vi "UNIX_Time.vi"(8 "error in (no error)":errorcluster) -> (0 "error out":errorcluster, 1 "Time zones addition":u32, 2 "Daylight savings subtraction":u32, 3 "Unix time - UTC":u32)   [LabVIEW 2013]
doc: "Outputs the current UNIX time (converts from the 1904 epoch LabVIEW based time to the 1970 UNIX epoch time). In addition, this VI takes into account the current time zone (and daylight saving settings) you have on your computer to get the accurate UNIX time conversion."
uses:
  kernel32.dll
panel:
  out "Timezoneinfotype":i32
  out "Sample UTC calc":u32
  out "Local time stamp":timestamp
  # "Seconds since midnight Jan 1st, 1970\nin UTC/GMT time"
  # "Hours"
  # "Hours"
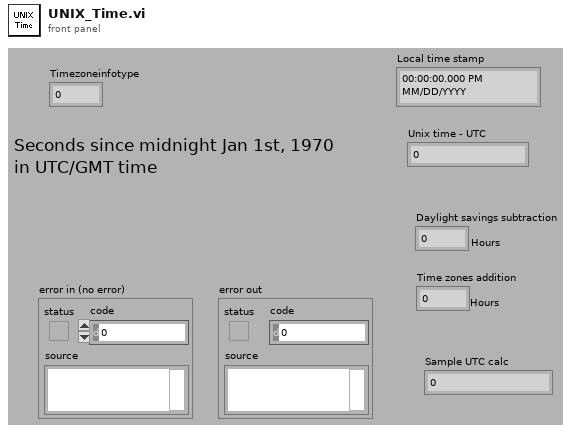
[diagram p1: front panel]
types:
  T1 = cluster{"[0]":u16, "[1]":u16, "[2]":u16, "[3]":u16, "[4]":u16, "[5]":u16, "[6]":u16, "[7]":u16, "[8]":u16, "[9]":u16, "[10]":u16, "[11]":u16, "[12]":u16, "[13]":u16, "[14]":u16, "[15]":u16, "[16]":u16, "[17]":u16, "[18]":u16, "[19]":u16, "[20]":u16, "[21]":u16, "[22]":u16, "[23]":u16, "[24]":u16, "[25]":u16, "[26]":u16, "[27]":u16, "[28]":u16, "[29]":u16, "[30]":u16, "[31]":u16, "[32]":u16, "[33]":u16, "[34]":u16, "[35]":u16, "[36]":u16, "[37]":u16, "[38]":u16, "[39]":u16, "[40]":u16, "[41]":u16, "[42]":u16, "[43]":u16, "[44]":u16, "[45]":u16, "[46]":u16, "[47]":u16, "[48]":u16, "[49]":u16, "[50]":u16, "[51]":u16, "[52]":u16, "[53]":u16, "[54]":u16, "[55]":u16, "[56]":u16, "[57]":u16, "[58]":u16, "[59]":u16, "[60]":u16, "[61]":u16, "[62]":u16, "[63]":u16, "[64]":u16, "[65]":u16, "[66]":u16, "[67]":u16, "[68]":u16, "[69]":u16, "[70]":u16, "[71]":u16, "[72]":u16, "[73]":u16, "[74]":u16, "[75]":u16, "[76]":u16, "[77]":u16, "[78]":u16, "[79]":u16, "[80]":u16, "[81]":u16, "[82]":u16, "[83]":u16, "[84]":u16, "[85]":u16}
  T2 = typedef "LVDateTimeRec.ctl" = cluster{"fractional second":dbl, "second":i32, "minute":i32, "hour":i32, "day of month":i32, "month":i32, "year":i32, "day of week":i32, "day of year":i32, "DST":i32}
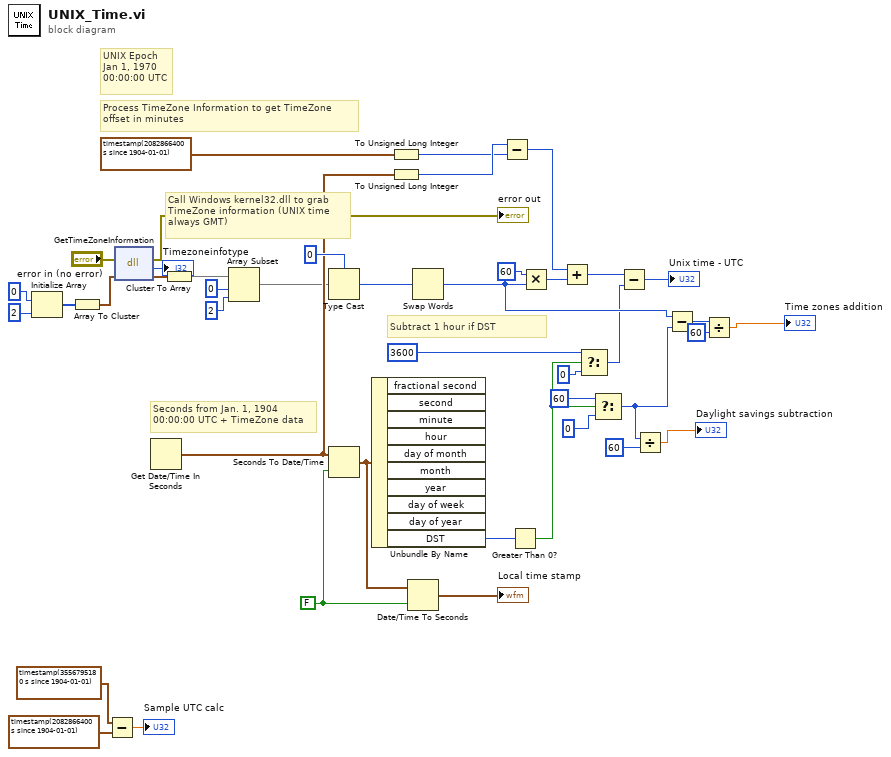
[diagram p0: block diagram]
diagram:
  w24 = FALSE ("to UTC (F)")
  # "Subtract 1 hour if DST"
  # "Seconds from Jan. 1, 1904\n00:00:00 UTC + TimeZone data"
  # "UNIX Epoch\nJan 1, 1970\n00:00:00 UTC"
  # "Process TimeZone Information to get TimeZone\noffset in minutes"
  # "Call Windows kernel32.dll to grab\nTimeZone information (UNIX time\nalways GMT)"
  n1 = Initialize Array(u16 0 ("element"), 2 ("dimension size")) -> (w40:u16[])
  n2 = Array To Cluster(array=w40) -> (cluster=w37:T1)
  n3 = Subtract(x=timestamp(3556795180 s since 1904-01-01), y=timestamp(2082866400 s since 1904-01-01)) -> (x-y=→"Sample UTC calc":dbl)
  n4 = dll-call lib="kernel32.dll" fn="GetTimeZoneInformation"(error in="error in (no error)", "lpTimeZoneInformation"=w37) -> (error out=→"error out":errorcluster, "return type"=→"Timezoneinfotype":i32, "lpTimeZoneInformation"=w36:T1)  [unwired: 2 in, 1 out]
  n5 = Get Date/Time In Seconds() -> (seconds since 1Jan1904=w20:timestamp)
  n6 = Cluster To Array(cluster=w36) -> (array=w35:u16[])
  n7 = Array Subset(array=w35, index=0, length=2) -> (w12:u16[])
  n8 = Type Cast(type=0, x=w12) -> (*(type *) &x=w31:i32)
  n9 = Seconds To Date/Time(time stamp (now)=w20, to UTC (F)=w24) -> (date time rec=w23:T2)
  n10 = Unbundle By Name(w23) -> ("DST"=w19:i32)  [unwired: 9 out]
  n11 = To Unsigned Long Integer(number=timestamp(2082866400 s since 1904-01-01)) -> (unsigned 32bit integer=w41:u32)
  n12 = To Unsigned Long Integer(number=w20) -> (unsigned 32bit integer=w42:u32)
  n13 = Date/Time To Seconds(1:w24, 2:w23) -> (0:→"Local time stamp":timestamp)
  n14 = Swap Words(1:w31) -> (0:w11:i32)
  n15 = Subtract(x=w42, y=w41) -> (x-y=w30:u32)
  n16 = Greater Than 0?(x=w19) -> (x > 0?=w9:bool)
  n17 = Multiply(x=u32 60 ("y"), y=w11) -> (x*y=w29:u32)
  n18 = Add(x=w30, y=w29) -> (x+y=w15:u32)
  n19 = Select(t=u32 3600, s=w9, f=u32 0) -> (s? t:f=w10:u32)
  n20 = Select(t=u32 60 ("f"), s=w9, f=u32 0) -> (s? t:f=w3:u32)
  n21 = Subtract(x=w15, y=w10) -> (x-y=→"Unix time - UTC":u32)
  n22 = Divide(x=w3, y=u32 60) -> (x/y=→"Daylight savings subtraction":dbl)
  n23 = Subtract(x=w11, y=w3) -> (x-y=w6:u32)
  n24 = Divide(x=w6, y=u32 60) -> (x/y=→"Time zones addition":dbl)
